vi "Set Default Overload Prot Tmo.vi"(8 "error in (no error)":errorcluster, 10 "Default Timeout Value (1.0 s)":dbl=1.0 format="%.4f", 11 "VISA resource name":refnum<visa-resource-name>) -> (0 "error out":errorcluster, 3 "VISA resource name out":refnum<visa-resource-name>)   [LabVIEW 2014, in "Fluke 5XXX Series Multicalibrators.lvlib"]
doc: "This VI sets the default OPERATE time limit for the OVERLD mode signal. The Calibrator automatically returns to STANDBY if the UUT protection trips within this interval or at the end of this interval if the protection has not tripped.\n\nNote:\n\nThis VI is available only for instrument models 5500A and 5520A with oscilloscope option SC600 (SC1100)."
uses:
  Fluke 5XXX Series Multicalibrators.lvlib
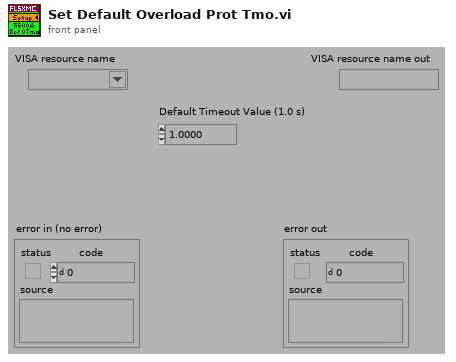
[diagram p1: front panel]
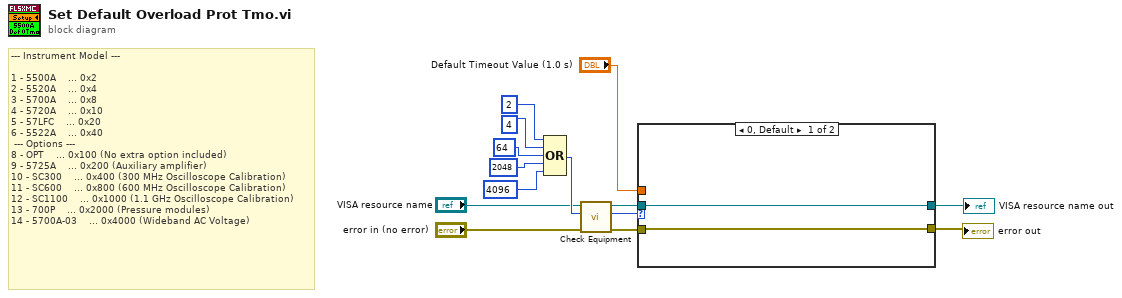
[diagram p0: block diagram]
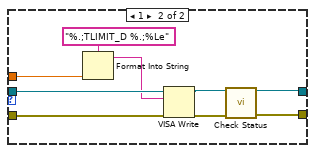
[diagram p2: hidden frame]
diagram:
  # "--- Instrument Model ---\n\n1 - 5500A    ... 0x2\n2 - 5520A    ... 0x4\n3 - 5700A    ... 0x8\n4 - 5720A    ... 0x10\n5 - 57LFC    ... 0x20\n6 - 5522A    ... 0x40\n --- Options ---\n8 - OPT    ... 0x100 (No extra option included)\n9 - 5725A    ... 0x200 (Auxiliary amplifier)\n10 - SC300    ... 0x400 (300 MHz Oscilloscope Calibration)\n11 - SC600    ... 0x800 (600 MHz Oscilloscope Calibration)\n12 - SC1100    ... 0x1000 (1.1 GHz Oscilloscope Calibration)\n13 - 700P    ... 0x2000 (Pressure modules)\n14 - 5700A-03    ... 0x4000 (Wideband AC Voltage)"
  n1 = Compound Arithmetic op=OR(2 ("Numeric"), 4 ("Numeric"), 64 ("Numeric"), 2048 ("Numeric"), 4096 ("Numeric")) -> (w7:i32)
  n2 = call "Check Equipment.vi"("error in (no error)"="error in (no error)", "Bit Mask"=w7, "VISA resource name"="VISA resource name") -> ("error out"=w14:errorcluster, "Present?"=w13:u32, "VISA resource name out"=w12:refnum<visa-resource-name>)  [unwired: 6 in]
  n3 = case shown="0, Default" w13 {
    tunnel: "Default Timeout Value (1.0 s)" -> [_ w17]
    tunnel: [w15 w20] -> w2
    tunnel: w14 -> [w16 w25]
    tunnel: w12 -> [w15 w24]
    tunnel: [w16 w23] -> w3
    frame 0, Default {
    }
    frame 1 {
      n4 = Format Into String(format string="%.;TLIMIT_D %.;%Le", w17) -> (resulting string=w18:string)  [unwired: 2 in, 1 out]
      n5 = VISA Write(VISA resource name=w24, write buffer=w18, error in (no error)=w25) -> (VISA resource name out=w21:refnum<visa-resource-name>, error out=w22:errorcluster)  [unwired: 1 out]
      n6 = call "Check Status.vi"("VISA resource name"=w21, "error in (no error)"=w22) -> ("VISA resource name out"=w20:refnum<visa-resource-name>, "error out"=w23:errorcluster)  [unwired: 12 in]
    }
  }
  "VISA resource name out" <- w2
  "error out" <- w3
